vi "loop.vi"() -> ()   [LabVIEW 2020]
uses:
  <vilib>/numeric/Random Number (Range) U64.vi
  <vilib>/numeric/sub_Random U32.vi
panel:
  in  "while/for":bool
  in  "stop":bool
  out "iteration num":dbl
  out "random num":dbl
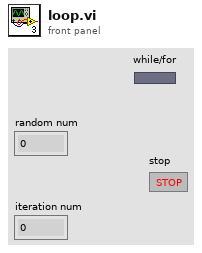
[diagram p1: front panel]
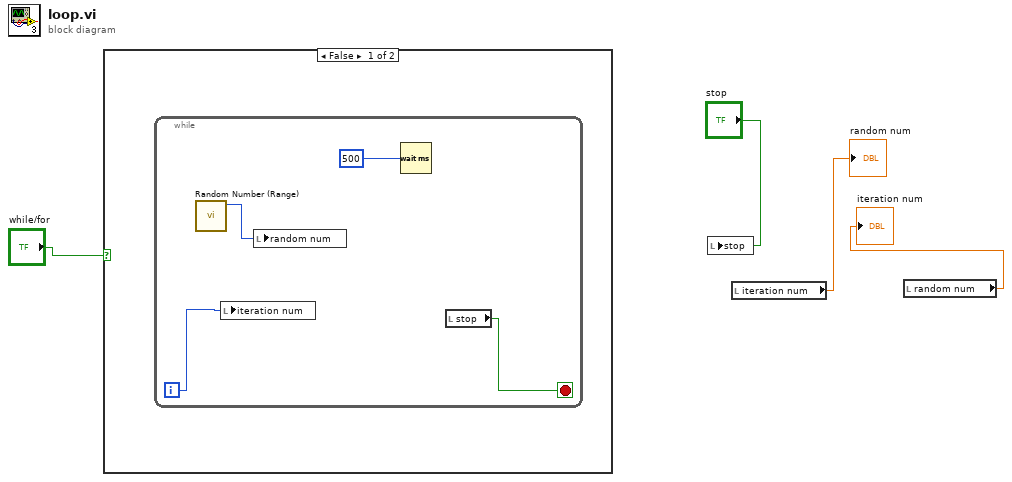
[diagram p0: block diagram]
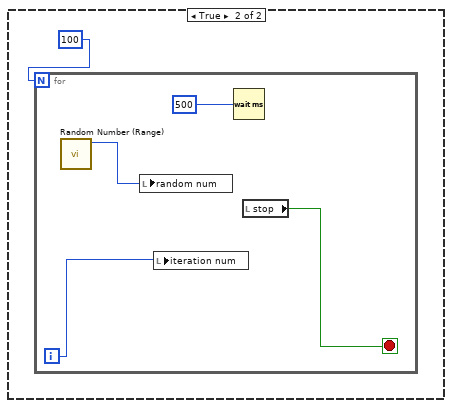
[diagram p2: hidden frame]
diagram:
  n1 = case shown="False" "while/for" {
    frame False {
      n2 = while {
        i -> [w6]
        stop <- w7 stop-if-true
        n3 = call-poly <vilib>:"Random Number (Range).vi"() -> ("number"=w5:u64)  [unwired: 11 in]
        n4 = local write "iteration num"(w6) -> ()
        n5 = local write "random num"(w5) -> ()
        n6 = Wait (ms)(milliseconds to wait=500) -> ()  [unwired: 1 out]
        n7 = local read "stop"() -> (w7:bool)
      }
    }
    frame True {
      n8 = for {
        N: 100 -> [_]
        i -> [w11]
        stop <- w12 stop-if-true
        n9 = call-poly <vilib>:"Random Number (Range).vi"() -> ("number"=w10:u64)  [unwired: 11 in]
        n10 = local write "random num"(w10) -> ()
        n11 = local write "iteration num"(w11) -> ()
        n12 = Wait (ms)(milliseconds to wait=500) -> ()  [unwired: 1 out]
        n13 = local read "stop"() -> (w12:bool)
      }
    }
  }
  n14 = local write "stop"("stop") -> ()
  n15 = local read "iteration num"() -> (→"random num":dbl)
  n16 = local read "random num"() -> (→"iteration num":dbl)
